vi "Real Time Display.vi"() -> ()   [LabVIEW 2015]
uses:
  Type/_Run Mode.ctl
  Type/_Data Operation.ctl
  Type/_RT Command.ctl
  Configuration/_Global Configuration.vi
  <vilib>/Utility/config.llb/Read Key (String).vi
  <vilib>/Utility/config.llb/Read Key (Double).vi
  <vilib>/Utility/config.llb/Read Key (I32).vi
  <vilib>/Utility/NIReport.llb/Append Image to Report (path wrap).vi
  <vilib>/Utility/NIReport.llb/NI_report.lvclass
  <vilib>/Utility/config.llb/NI_LVConfig.lvlib
panel:
  out "error out 2":errorcluster
  out "error out":errorcluster
  in  "Comments":string
  out "Close":bool
  out "Q2DC POL":bool
  out "Q1DC POL":bool
  out "Date":string
  out "MCA":bool
  out "Run Mode":T1
  out "Q2 Resolution":i32[](listbox) caption="Q2 +ve High Res"
  out "Q1 Resolution":i32[](listbox) caption="Q1 +ve High Res"
  out "Q2 Calibration":i32[](listbox)
  out "Q1 Calibration":i32[](listbox)
  out "Scan #":i32=1
  out "Peak List":i32[](listbox)
  out "Lens Values":i32[](listbox)
  out "TIC":cluster{"TIC X":dbl[], "TIC Y":dbl[]}[](graph)
  out "Run Time":i32=1 caption="Run Time (ms)"
  in  "Expt#":i32=1 caption="Experiment #"
  out "Init":bool
  out "A 6":bool
  out "A 5":bool
  out "A 4":bool
  out "A 3":bool
  out "A 2":bool
  out "A 1":bool
  out "MR 5":cluster{dbl[], dbl[]}(graph)
  out "MR 4":cluster{dbl[], dbl[]}(graph)
  out "MR 2":cluster{dbl[], dbl[]}(graph)
  out "MR 1":cluster{dbl[], dbl[]}(graph)
  out "MR 6":cluster{dbl[], dbl[]}(graph)
  out "MR 3":cluster{dbl[], dbl[]}(graph)
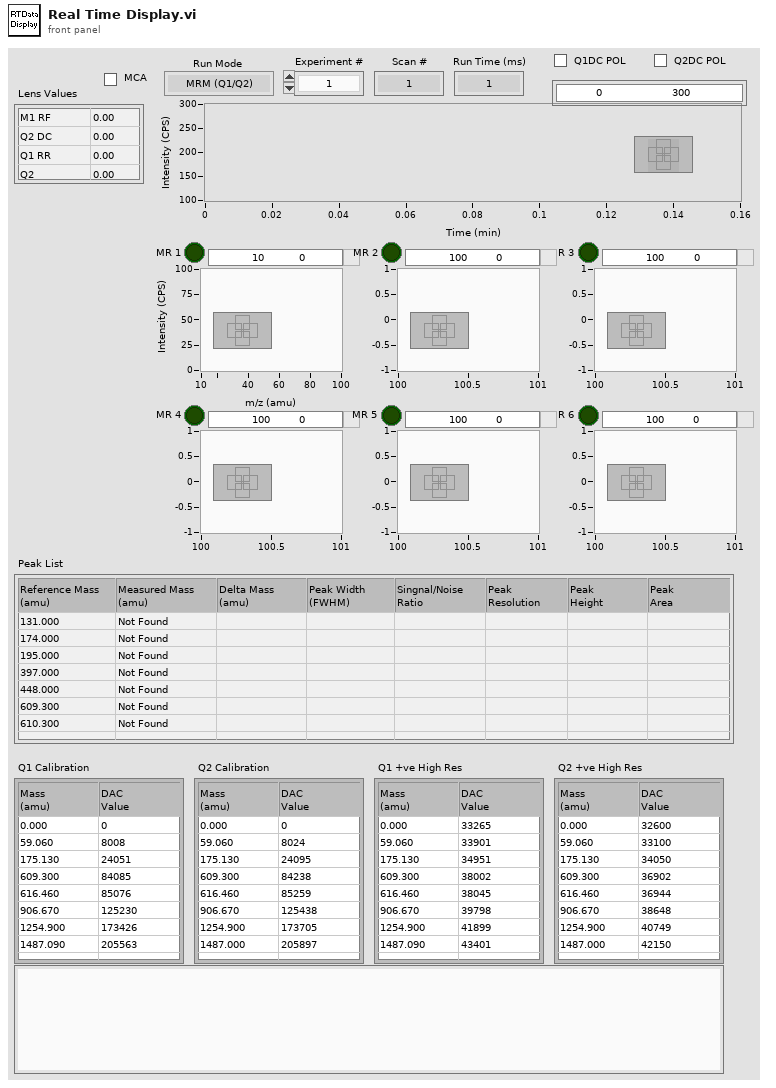
[diagram p1: front panel]
types:
  T1 = typedef "_Run Mode.ctl" = enum16{"MRM (Q1/Q2)", "Q1 Scan", "Q1 SRM", "Q2 Scan", "Q2 SRM", "Product Scan", "Precursor Scan", "Neutral Loss", "Neutral Gain"}
  T2 = cluster{"TIC":refnum<vi>, "MR 1":refnum<vi>, "MR 2":refnum<vi>, "MR 3":refnum<vi>, "MR 4":refnum<vi>, "MR 5":refnum<vi>, "MR 6":refnum<vi>, "A 1":refnum<vi>, "A 2":refnum<vi>, "A 3":refnum<vi>, "A 4":refnum<vi>, "A 5":refnum<vi>, "A 6":refnum<vi>, "Lens Values":refnum<vi>, "Q1 Calibration":refnum<vi>, "Q2 Calibration":refnum<vi>, "Q1 Resolution":refnum<vi>, "Q2 Resolution":refnum<vi>, "Peak List":refnum<vi>, "Comments":refnum<vi>}
  T3 = cluster{"RefMass":dbl[], "LensList":i32[], "SearchWin":dbl, "MinH":dbl, "MinW":i32, "RunTime":i32}
  T4 = enum16{"Standard Report", "HTML", "Word", "Excel"}
  T5 = typedef "_Data Operation.ctl" = enum8{"Initialize", "Get Data", "Set Data", "Close"}
  T6 = typedef "_RT Command.ctl" = enum16{"xml Start Run", "xml Start Actual Run", "xml Stop Run", "xml Runtime Update", "xml Get Status", "xml Get Table", "xml Set Table", "xml Get Configuration", "xml System Status", "xml Set LC Input Logic", "xml Get Data", "xml Get Info", "Start", "StartActualRun", "Stop", "Runtime Update", "Get Data", "Get Info", "Get Status", "Get Param", "Get Config", "Get Table", "Read ADC", "Set Oscillator", "Update Config", "Update Table", "Set All Pol", "Set Pol and DC", "Set Max Mass", "Toggle RP", "Toggle EL", "Set PIC", "Initialize Turbo", "Send Turbo Comm", "Close Turbo", "P1", "P2", "P3", "Send Serial", "Set LC Out", "Get LC In", "Read VAC", "Test Table", "Toggle Power", "Get Startup", "Set Startup", "Get ADC Table", "Set ADC Table", "Get Brief Status", "Get Detail Status", "Auxiliary Update", "Set CC Logics", "Set CC Input Logics", "Ignore Error", "invalid"}
  T7 = typedef "NI_LVConfig.lvlib/Config Data RefNum.ctl" = refnum<k1>
  T8 = typedef "_Current Data.ctl" = cluster{"Scan#":i32, "Run Time (mS)":i32, "TIC X":dbl[], "TIC Y":dbl[][], "MassRange":cluster{"X Title":string, "X":dbl[], "Y":i32[]}[], "Fixed Mass (amu)":dbl, "Method":T9}
  T9 = typedef "_XML Expt.ctl" = cluster{"StartT(mS)":i32, "#Cycles":i32, "PauseT(uS)":i32, "ScanType":i32, "Polarity":u8, "FixedMass":dbl, "DelayT(mS)":i32, "Active Ch":T10[], "Mass Range":T11[]}
  T10 = typedef "_XML Lens.ctl" = cluster{"Value":dbl, "ChID":u8}
  T11 = typedef "_Mass Range Property.ctl" = cluster{"Start":dbl, "Stop":dbl, "Step Size":dbl, "Steps":i32, "Dwell":dbl, "Parameters":T12[], "Res":T13}
  T12 = typedef "_Mass Range Parameters.ctl" = cluster{"Name":string, "Ch#":u8, "StartV":dbl, "StopV":dbl, "StepV":dbl, "Index":u8}
  T13 = typedef "_RT Res Type.ctl" = u16
  T14 = typedef "_Peak Property.ctl" = cluster{"Centroid":dbl, "Height":dbl, "FWHM":dbl, "Resolution":dbl, "Area":dbl, "StoN":dbl, "ApexX":dbl, "Baseline":dbl, "LEdgeX":dbl, "LEdgeY":dbl, "REdgeX":dbl, "REdgeY":dbl, "LEdgeFWHM":dbl, "REdgeFWHM":dbl}
  T15 = typedef "imagedata.ctl" = cluster{"image type":i32, "image depth":i32, "image":u8[], "mask":u8[], "colors":u32[], "Rectangle":cluster{"left":i16, "top":i16, "right":i16, "bottom":i16}}
  T16 = typedef "LVRangeTypeDef.ctl" = cluster{"Minimum":dbl, "Maximum":dbl, "Increment":dbl, "Minor Increment":dbl, "Start":dbl}
  T17 = typedef "LVPointDoubleTypeDef.ctl" = cluster{"Cursor X":dbl, "Cursor Y":dbl}
  T18 = cluster{"YScale.NameLbl.Text":string, "XScale.NameLbl.Text":string, "XScale.Range":T16, "YScale.Range":T16, "Label.Text":string, "Cursor.Cursor Position":T17, "Plot.Bar Plot Style":u8}
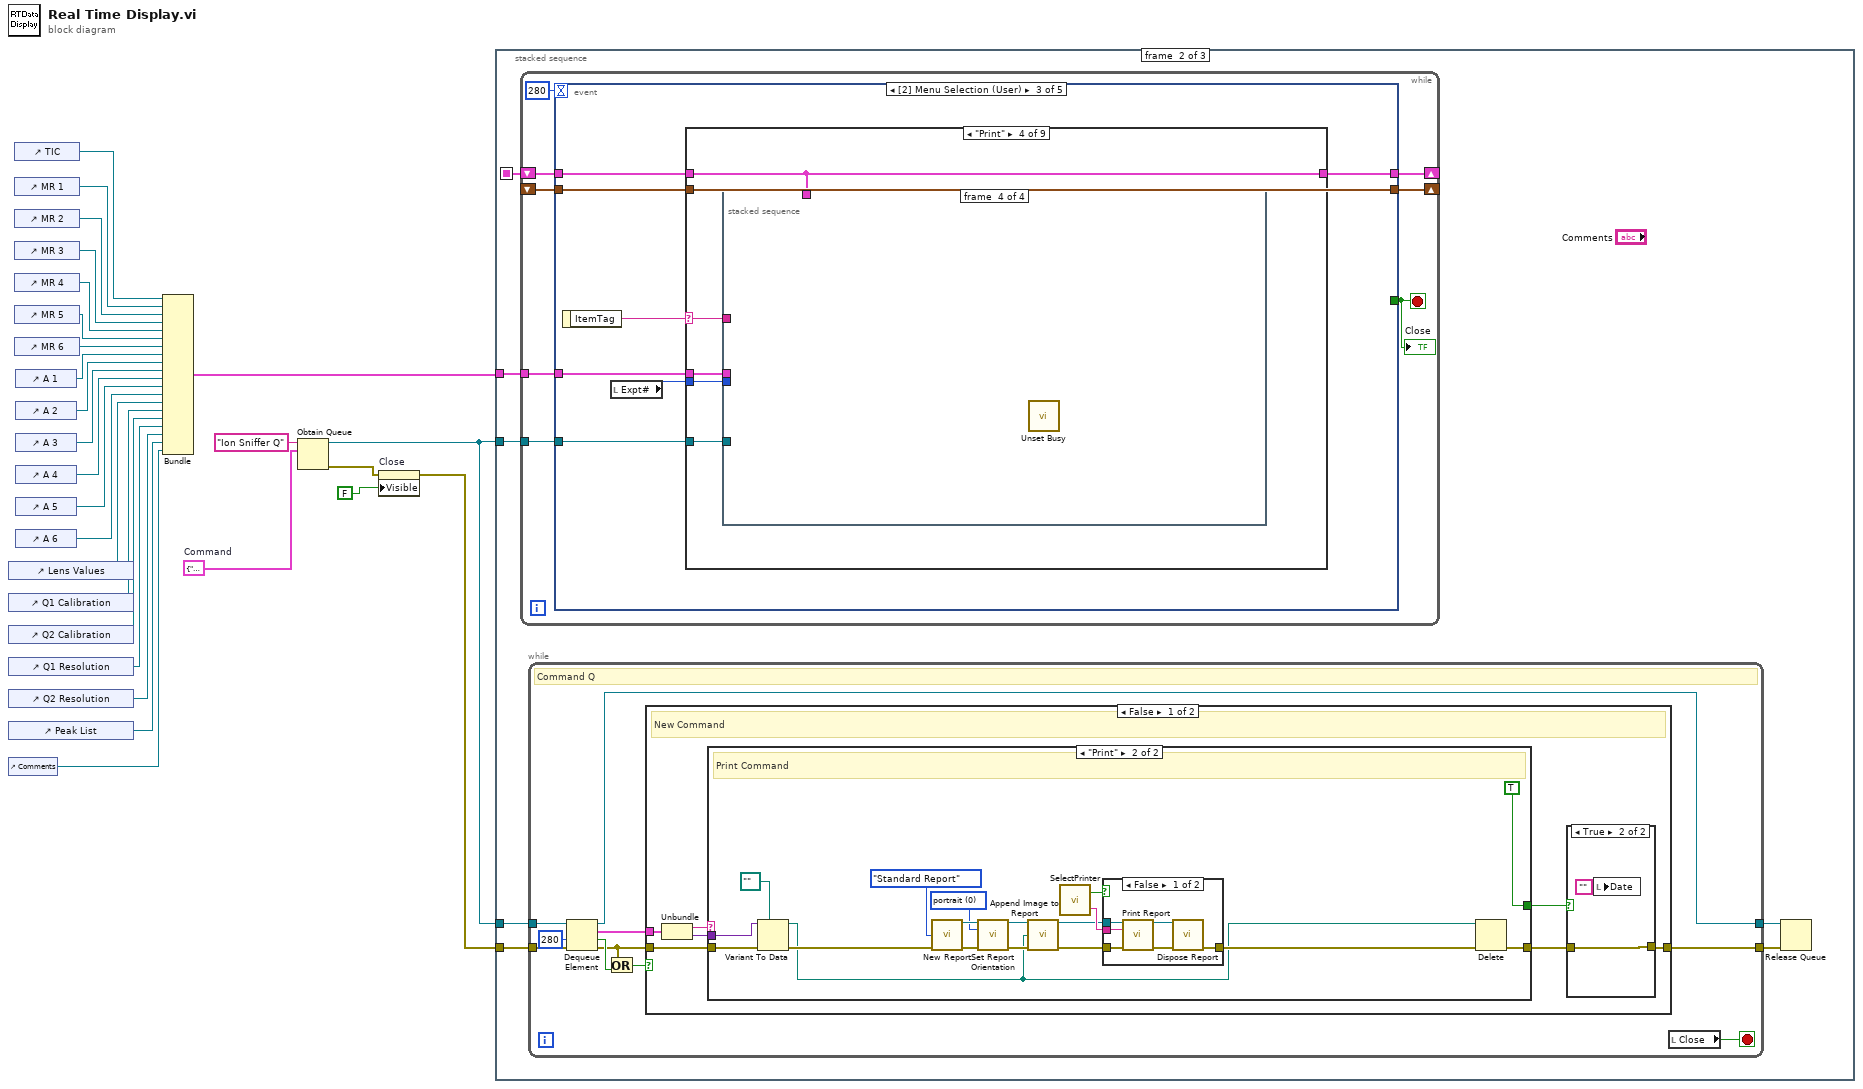
[diagram p0: block diagram]
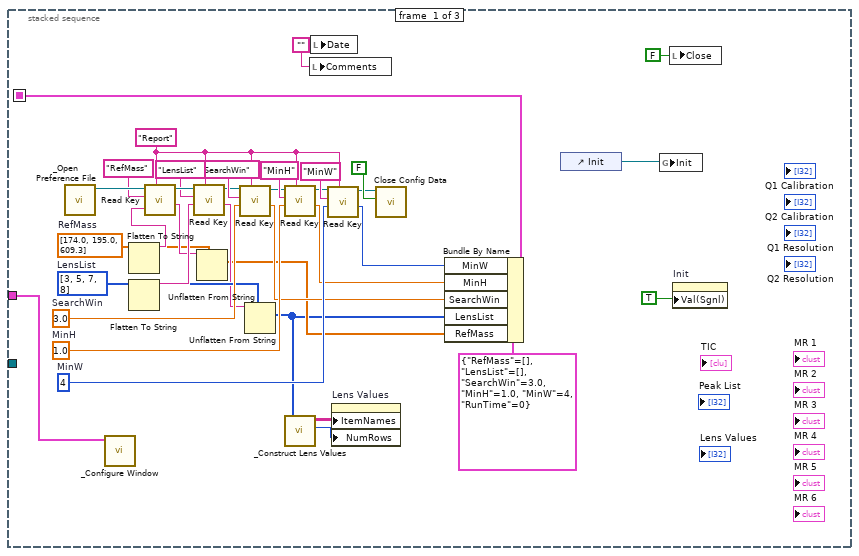
[diagram p2: hidden frame]
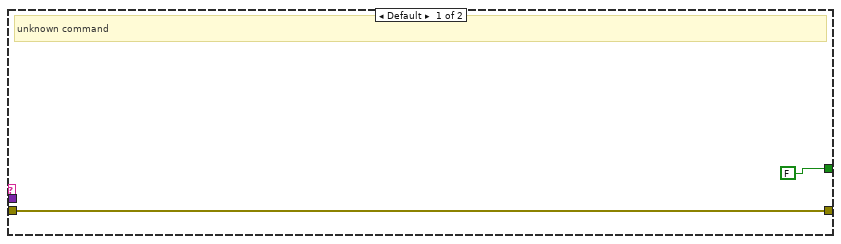
[diagram p4: hidden frame]
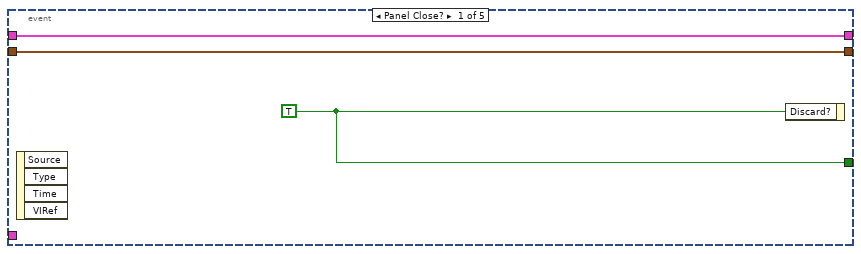
[diagram p7: hidden frame]
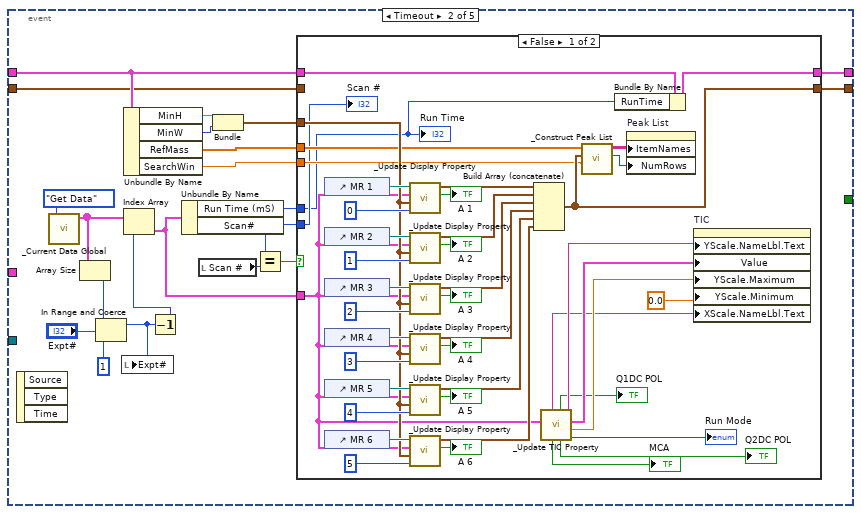
[diagram p8: hidden frame]
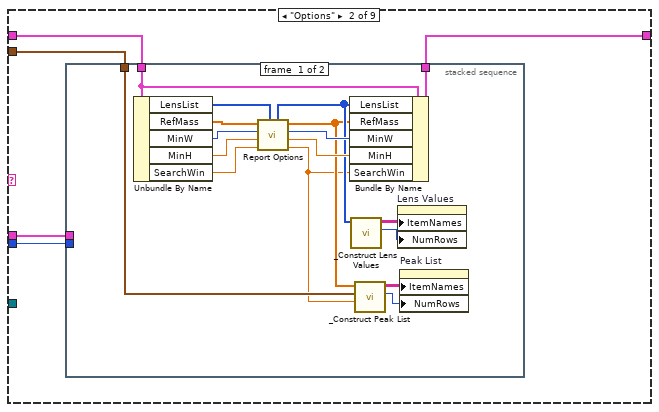
[diagram p11: hidden frame]
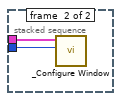
[diagram p12: hidden frame]
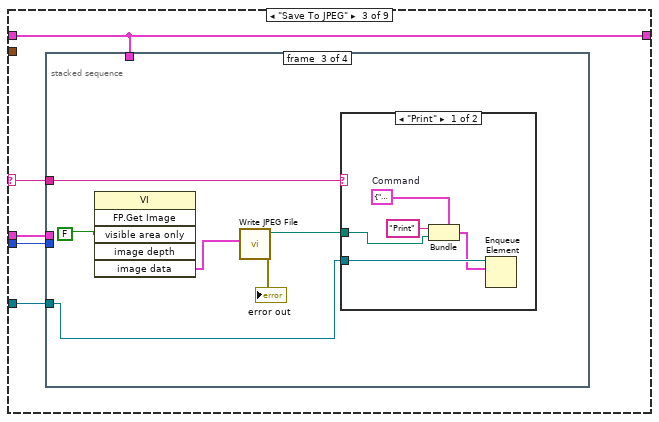
[diagram p13: hidden frame]
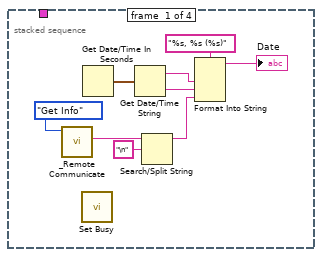
[diagram p14: hidden frame]
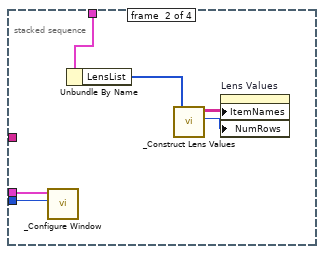
[diagram p15: hidden frame]
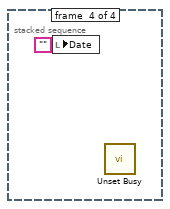
[diagram p17: hidden frame]
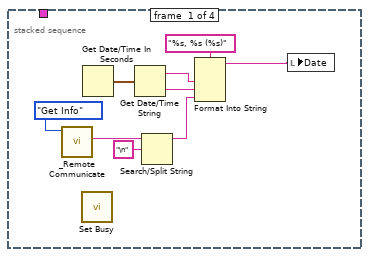
[diagram p18: hidden frame]
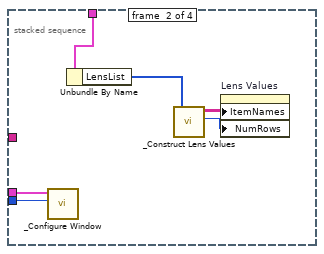
[diagram p19: hidden frame]
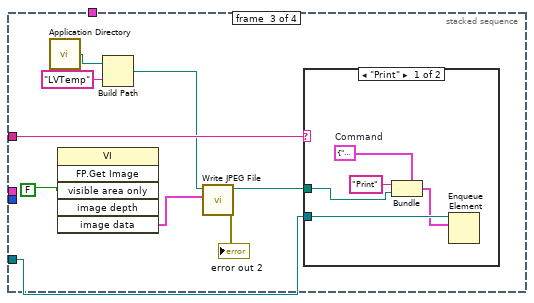
[diagram p20: hidden frame]
diagram:
  w1 = cluster{"Command":string, "Data":variant} {"Command"="", "Data"=variant}  # Command
  n1 = control-ref of="Lens Values"() -> (w27:refnum<vi>)
  n2 = control-ref of="Q1 Calibration"() -> (w13:refnum<vi>)
  n3 = control-ref of="Q2 Calibration"() -> (w12:refnum<vi>)
  n4 = control-ref of="Q1 Resolution"() -> (w11:refnum<vi>)
  n5 = control-ref of="Q2 Resolution"() -> (w10:refnum<vi>)
  n6 = control-ref of="Peak List"() -> (w9:refnum<vi>)
  n7 = control-ref of="Comments"() -> (w2:refnum<vi>)
  n8 = control-ref of="TIC"() -> (w8:refnum<vi>)
  n9 = control-ref of="MR 1"() -> (w15:refnum<vi>)
  n10 = control-ref of="MR 2"() -> (w16:refnum<vi>)
  n11 = control-ref of="MR 3"() -> (w17:refnum<vi>)
  n12 = control-ref of="MR 4"() -> (w18:refnum<vi>)
  n13 = control-ref of="MR 5"() -> (w19:refnum<vi>)
  n14 = control-ref of="MR 6"() -> (w20:refnum<vi>)
  n15 = control-ref of="A 1"() -> (w21:refnum<vi>)
  n16 = control-ref of="A 2"() -> (w22:refnum<vi>)
  n17 = control-ref of="A 3"() -> (w23:refnum<vi>)
  n18 = control-ref of="A 4"() -> (w24:refnum<vi>)
  n19 = control-ref of="A 5"() -> (w25:refnum<vi>)
  n20 = control-ref of="A 6"() -> (w26:refnum<vi>)
  n21 = Bundle("TIC"=w8, "MR 1"=w15, "MR 2"=w16, "MR 3"=w17, "MR 4"=w18, "MR 5"=w19, "MR 6"=w20, "A 1"=w21, "A 2"=w22, "A 3"=w23, "A 4"=w24, "A 5"=w25, "A 6"=w26, "Lens Values"=w27, "Q1 Calibration"=w13, "Q2 Calibration"=w12, "Q1 Resolution"=w11, "Q2 Resolution"=w10, "Peak List"=w9, "Comments"=w2) -> (w14:T2)  [unwired: 1 out]
  n22 = Obtain Queue(name (unnamed)="Ion Sniffer Q", element data type=w1) -> (queue out=w6:refnum<queue>, error out=w4:errorcluster)  [unwired: 3 in, 1 out]
  n23 = property on="Close" class="Bool (strict)"(error in=w4, "Visible"=FALSE) -> (error out=w5:errorcluster)  [unwired: 1 in, 1 out]
  n24 = stacked-sequence {
    seq-local: [w34 _ _] -> [_ w70 _]
    tunnel: w14 -> [w30 w69 _]
    tunnel: w6 -> [_ w68 _]
    tunnel: w6 -> [_ w67 _]
    tunnel: w5 -> [_ w66 _]
    frame #0 {
      w28 = ""
      w50 = "Report" ("section")
      w41 = i32[] [3, 5, 7, 8]  # LensList
      w46 = 4  # MinW
      w47 = 1.0  # MinH
      w48 = 3.0  # SearchWin
      w42 = dbl[] [174.0, 195.0, 609.3]  # RefMass
      n25 = call "_Open Preference File.vi"() -> ("refnum"=w59:T7)  [unwired: 3 in, 4 out]
      n26 = call "_Configure Window.vi"("ControlRef"=w30) -> ()  [unwired: 2 in, 5 out]
      n27 = Flatten To String(anything=w42) -> (data string=w45:string)  [unwired: 1 in, 4 out]
      n28 = Flatten To String(anything=w41) -> (data string=w44:string)  [unwired: 1 in, 4 out]
      n29 = call-poly <vilib>:"Read Key.vi"("section"=w50, "default value"=w45, "key"="RefMass", "refnum"=w59) -> ("value"=w43:string, "refnum out"=w61:T7)  [unwired: 2 in, 4 out]
      n30 = call-poly <vilib>:"Read Key.vi"("section"=w50, "default value"=w44, "key"="LensList" ("section"), "refnum"=w61) -> ("value"=w40:string, "refnum out"=w53:T7)  [unwired: 2 in, 4 out]
      n31 = Unflatten From String(type=w42, binary string=w43) -> (value=w35:dbl[])  [unwired: 1 in, 4 out]
      n32 = call-poly <vilib>:"Read Key.vi"("section"=w50, "default value"=w48, "key"="SearchWin", "refnum"=w53) -> ("value"=w36:dbl, "refnum out"=w54:T7)  [unwired: 1 in, 5 out]
      n33 = Unflatten From String(type=w41, binary string=w40) -> (value=w33:i32[])  [unwired: 1 in, 4 out]
      n34 = call-poly <vilib>:"Read Key.vi"("section"=w50, "default value"=w47, "key"="MinH" ("section"), "refnum"=w54) -> ("value"=w37:dbl, "refnum out"=w51:T7)  [unwired: 1 in, 5 out]
      n35 = call "_Construct Lens Values.vi"("Lens List"=w33) -> ("# of Lens"=w31:i32, "Table"=w32:string[][])  [unwired: 5 out]
      n36 = local write "Comments"(w28) -> ()
      n37 = local write "Date"(w28) -> ()
      n38 = call-poly <vilib>:"Read Key.vi"("section"=w50, "default value"=w46, "key"="MinW" ("section"), "refnum"=w51) -> ("value"=w38:i32, "refnum out"=w49:T7)  [unwired: 1 in, 5 out]
      n39 = property on="Lens Values" class="MCListbox (strict)"("ItemNames"=w32, "NumRows"=w31) -> ()  [unwired: 2 in, 2 out]
      n40 = call <vilib>:"Close Config Data.vi"("write file if changed (T)"=FALSE ("write configuration file? (F)"), "refnum"=w49) -> ()  [unwired: 1 in, 9 out]
      n41 = Bundle By Name(cluster=T3 {"RefMass"=[], "LensList"=[], "SearchWin"=3.0, "MinH"=1.0, "MinW"=4, "RunTime"=0}, "MinW"=w38, "MinH"=w37, "SearchWin"=w36, "LensList"=w33, "RefMass"=w35) -> (w34:T3)
      n42 = control-ref of="Init"() -> (w63:refnum<vi>)
      n43 = global write "_Global Configuration.vi" "Init"(w63) -> ()
      n44 = local write "Close"(FALSE ("Close")) -> ()
      n45 = property on="Init" class="Bool (strict)"("Val(Sgnl)"=TRUE ("Value (Signaling)")) -> ()  [unwired: 2 in, 2 out]
    }
    frame #1 {
      n46 = while {
        shift-right: [w125] -> _
        shift-left: w70 -> [w126]
        shift-right: [w124] -> _
        shift-left: _ -> [w123]
        tunnel: w69 -> [w122]
        tunnel: w68 -> [w120]
        stop <- w119 stop-if-true
        n47 = event shown="[2] Menu Selection (User)" {
          selector: _ -> [_ _ _ _ _]
          dyn-events: _ -> [_ _ _ _ _]
          timeout: 280 -> [_ _ _ _ _]
          tunnel: [w129 _ _ _ _] -> w119
          tunnel: w126 -> [w128 w150 w202 w322 w328]
          tunnel: [w128 w149 w201 w323 w328] -> w125
          tunnel: [w127 w147 w200 w318 w327] -> w124
          tunnel: w123 -> [w127 w148 w200 w318 w327]
          tunnel: w122 -> [_ _ w199 w316 _]
          tunnel: w120 -> [_ _ w197 _ _]
          event Panel Close? {
            w129 = TRUE ("Discard?")
            n48 = event-data() -> ()  [unwired: 5 out]
            n49 = event-data("Discard?"=w129) -> ()  [unwired: 1 in, 1 out]
          }
          event Timeout {
            n50 = event-data() -> ()  [unwired: 4 out]
            n51 = call "_Current Data Global.vi"("Operation"=_Data_Operation."Get Data") -> ("CurrentData"=w139:T8[])  [unwired: 3 in, 3 out]
            n52 = Array Size(array=w139) -> (size(s)=w136:i32)
            n53 = In Range and Coerce(upper limit=w136, x="Expt#", lower limit=1) -> (coerced(x)=w135:i32)  [unwired: 1 out]
            n54 = local write "Expt#"(w135) -> ()
            n55 = Unbundle By Name(w150) -> ("MinH"=w145:dbl, "MinW"=w144:i32, "RefMass"=w142:dbl[], "SearchWin"=w141:dbl)
            n56 = Decrement(x=w135) -> (x-1=w134:i32)
            n57 = Index Array(array=w139, index=w134) -> (element=w140:T8)
            n58 = Unbundle By Name(w140) -> ("Run Time (mS)"=w130:i32, "Scan#"=w132:i32)
            n59 = local read "Scan #"() -> (w133:i32)
            n60 = Bundle("MinH"=w145, "MinW"=w144) -> (w143:cluster{"MinH":dbl, "MinW":i32})  [unwired: 1 out]
            n61 = Equal?(x=w132, y=w133) -> (x = y?=w131:bool)
            n62 = case shown="False" w131 {
              tunnel: w150 -> [w194 w196]
              tunnel: [w193 w196] -> w149
              tunnel: [w165 w195] -> w147
              tunnel: w148 -> [_ w195]
              tunnel: w143 -> [w179 _]
              tunnel: w140 -> [w161 _]
              tunnel: w142 -> [w164 _]
              tunnel: w141 -> [w163 _]
              tunnel: w132 -> [w162 _]
              tunnel: w130 -> [w154 _]
              frame False {
                n63 = control-ref of="MR 1"() -> (w192:refnum<vi>)
                n64 = control-ref of="MR 2"() -> (w191:refnum<vi>)
                n65 = control-ref of="MR 3"() -> (w189:refnum<vi>)
                n66 = control-ref of="MR 4"() -> (w187:refnum<vi>)
                n67 = control-ref of="MR 5"() -> (w185:refnum<vi>)
                n68 = control-ref of="MR 6"() -> (w183:refnum<vi>)
                n69 = call "_Update Display Property.vi"("MassRange# (0)"=0, "PeakParam"=w179, "Current Data"=w161, "Display Refnum"=w192) -> ("Active"=→"A 1":bool, "Peak List"=w173:T14[])  [unwired: 3 out]
                n70 = call "_Update Display Property.vi"("MassRange# (0)"=1, "PeakParam"=w179, "Current Data"=w161, "Display Refnum"=w191) -> ("Active"=→"A 2":bool, "Peak List"=w172:T14[])  [unwired: 3 out]
                n71 = call "_Update Display Property.vi"("MassRange# (0)"=2, "PeakParam"=w179, "Current Data"=w161, "Display Refnum"=w189) -> ("Active"=→"A 3":bool, "Peak List"=w171:T14[])  [unwired: 3 out]
                n72 = call "_Update Display Property.vi"("MassRange# (0)"=3, "PeakParam"=w179, "Current Data"=w161, "Display Refnum"=w187) -> ("Active"=→"A 4":bool, "Peak List"=w170:T14[])  [unwired: 3 out]
                n73 = call "_Update Display Property.vi"("MassRange# (0)"=4, "PeakParam"=w179, "Current Data"=w161, "Display Refnum"=w185) -> ("Active"=→"A 5":bool, "Peak List"=w169:T14[])  [unwired: 3 out]
                n74 = call "_Update Display Property.vi"("MassRange# (0)"=5, "PeakParam"=w179, "Current Data"=w161, "Display Refnum"=w183) -> ("Active"=→"A 6":bool, "Peak List"=w168:T14[])  [unwired: 3 out]
                n75 = Build Array (concatenate)(w173, w172, w171, w170, w169, w168) -> (w165:T14[])
                n76 = call "_Update TIC Property.vi"("Current Data"=w161) -> ("Run Mode"=→"Run Mode":T1, "YMax"=w158:dbl, "TIC Data"=w159:cluster{"TIC X":dbl[], "Data in cps":dbl[]}[], "YTitle"=w160:string, "Q2DC Pol"=→"Q2DC POL":bool, "Q1DC Pol"=→"Q1DC POL":bool, "MCA"=→"MCA":bool, "XTitle"=w153:string)  [unwired: 3 out]
                n77 = call "_Construct Peak List.vi"("Search Window"=w163, "Peak List"=w165, "RefMass"=w164) -> ("# of Peaks"=w166:i32, "Table"=w167:string[][])  [unwired: 3 out]
                n78 = Bundle By Name(cluster=w194, "RunTime"=w154) -> (w193:T3)
                n79 = property on="Peak List" class="MCListbox (strict)"("ItemNames"=w167, "NumRows"=w166) -> ()  [unwired: 2 in, 2 out]
                n80 = property on="TIC" class="XYGraph (strict)"("YScale.NameLbl.Text"=w160, "Value"=w159, "YScale.Maximum"=w158, "YScale.Minimum"=0.0 ("Y Scale.Range:Minimum"), "XScale.NameLbl.Text"=w153) -> ()  [unwired: 2 in, 2 out]
                "Run Time" <- w154
                "Scan #" <- w162
              }
              frame True {
              }
            }
          }
          event Menu Selection (User) {
            n81 = event-data() -> ("ItemTag"=w203:string)  [unwired: 1 out]
            n82 = local read "Expt#"() -> (w198:i32)
            n83 = case shown="\"Print\"" w203 {
              selector: w203 -> [_ _ w230 w262 _ _ _ _ _]
              tunnel: w202 -> [w204 w209 w233 w265 w297 w298 w301 w303 w315]
              tunnel: [w204 w208 w233 w265 w297 w298 w301 w303 w315] -> w201
              tunnel: w200 -> [_ w207 _ _ w296 _ _ _ _]
              tunnel: w199 -> [_ w206 w232 w264 _ _ _ w304 w314]
              tunnel: w198 -> [_ w205 w231 w263 _ _ _ w302 w313]
              tunnel: w197 -> [_ _ w229 w261 _ _ _ _ _]
              frame Default {
              }
              frame "Options" {
                n84 = stacked-sequence {
                  tunnel: w209 -> [w210 _]
                  tunnel: [w221 _] -> w208
                  tunnel: w207 -> [w218 _]
                  tunnel: w206 -> [_ w228]
                  tunnel: w205 -> [_ w227]
                  frame #0 {
                    n85 = Unbundle By Name(w210) -> ("LensList"=w226:i32[], "RefMass"=w217:dbl[], "MinW"=w225:i32, "MinH"=w224:dbl, "SearchWin"=w216:dbl)
                    n86 = call "Report Options.vi"("LensList"=w226, "Search Window"=w216, "Min. Height"=w224, "Min. Width"=w225, "RefMass"=w217) -> ("Search Window 2"=w211:dbl, "Min. Height 2"=w222:dbl, "Min. Width 2"=w223:i32, "RefMass 2"=w212:dbl[], "LensList 2"=w213:i32[])
                    n87 = Bundle By Name(cluster=w210, "LensList"=w213, "RefMass"=w212, "MinW"=w223, "MinH"=w222, "SearchWin"=w211) -> (w221:T3)
                    n88 = call "_Construct Lens Values.vi"("Lens List"=w213) -> ("# of Lens"=w214:i32, "Table"=w215:string[][])  [unwired: 5 out]
                    n89 = call "_Construct Peak List.vi"("Search Window"=w211, "Peak List"=w218, "RefMass"=w212) -> ("# of Peaks"=w219:i32, "Table"=w220:string[][])  [unwired: 3 out]
                    n90 = property on="Lens Values" class="MCListbox (strict)"("ItemNames"=w215, "NumRows"=w214) -> ()  [unwired: 2 in, 2 out]
                    n91 = property on="Peak List" class="MCListbox (strict)"("ItemNames"=w220, "NumRows"=w219) -> ()  [unwired: 2 in, 2 out]
                  }
                  frame #1 {
                    n92 = call "_Configure Window.vi"("Expt#"=w227, "ControlRef"=w228) -> ()  [unwired: 1 in, 5 out]
                  }
                }
              }
              frame "Save To JPEG" {
                n93 = stacked-sequence {
                  tunnel: w233 -> [_ w246 _ _]
                  tunnel: w232 -> [_ w244 _ _]
                  tunnel: w231 -> [_ w243 _ _]
                  tunnel: w230 -> [_ _ w252 _]
                  tunnel: w229 -> [_ _ w249 _]
                  frame #0 {
                    n94 = call "_Remote Communicate.vi"("Command"=_RT_Command."Get Info") -> ("Info"=w241:string)  [unwired: 5 in, 3 out]
                    n95 = call <vilib>:"Set Busy.vi"() -> ()  [unwired: 4 in, 8 out]
                    n96 = Get Date/Time In Seconds() -> (seconds since 1Jan1904=w239:timestamp)
                    n97 = Get Date/Time String(seconds (now)=w239) -> (date string=w237:string, time string=w236:string)  [unwired: 2 out]
                    n98 = Search/Split String(string=w241, search string/char (-)="\n") -> (substring before match=w235:string)  [unwired: 3 out]
                    n99 = Format Into String(format string="%s, %s (%s)", w237, w236, w235) -> (resulting string=→"Date":string)  [unwired: 2 in, 1 out]
                  }
                  frame #1 {
                    n100 = call "_Configure Window.vi"("Expt#"=w243, "ControlRef"=w244) -> ()  [unwired: 1 in, 5 out]
                    n101 = Unbundle By Name(w246) -> ("LensList"=w245:i32[])
                    n102 = call "_Construct Lens Values.vi"("Lens List"=w245) -> ("# of Lens"=w247:i32, "Table"=w248:string[][])  [unwired: 5 out]
                    n103 = property on="Lens Values" class="MCListbox (strict)"("ItemNames"=w248, "NumRows"=w247) -> ()  [unwired: 2 in, 2 out]
                  }
                  frame #2 {
                    n104 = invoke class="VI" method="FP.Get Image"("visible area only"=FALSE ("Visible Area Only")) -> ("image data"=w253:T15)  [unwired: 5 in, 5 out]
                    n105 = call <vilib>:"Write JPEG File.vi"("image data"=w253) -> ("error out"=→"error out":errorcluster, "path"=w251:path)  [unwired: 2 in, 7 out]
                    n106 = case shown="\"Print\"" w252 {
                      tunnel: w251 -> [w255 _]
                      tunnel: w249 -> [w259 _]
                      frame "Print" {
                        w258 = cluster{"Command":string, "Data":variant} {"Command"="", "Data"=variant}  # Command
                        n107 = Bundle(cluster=w258, "Command"="Print", "Data"=w255) -> (w256:cluster{"Command":string, "Data":variant})
                        n108 = Enqueue Element(queue=w259, element=w256) -> ()  [unwired: 2 in, 3 out]
                      }
                      frame Default {
                      }
                    }
                  }
                  frame #3 {
                    n109 = local write "Date"("") -> ()
                    n110 = call <vilib>:"Unset Busy.vi"() -> ()  [unwired: 2 in, 10 out]
                  }
                }
              }
              frame "Print" {
                n111 = stacked-sequence {
                  tunnel: w265 -> [_ w278 _ _]
                  tunnel: w264 -> [_ w276 _ _]
                  tunnel: w263 -> [_ w275 _ _]
                  tunnel: w262 -> [_ _ w287 _]
                  tunnel: w261 -> [_ _ w284 _]
                  frame #0 {
                    n112 = call "_Remote Communicate.vi"("Command"=_RT_Command."Get Info") -> ("Info"=w273:string)  [unwired: 5 in, 3 out]
                    n113 = call <vilib>:"Set Busy.vi"() -> ()  [unwired: 4 in, 8 out]
                    n114 = Get Date/Time In Seconds() -> (seconds since 1Jan1904=w271:timestamp)
                    n115 = Get Date/Time String(seconds (now)=w271) -> (date string=w269:string, time string=w268:string)  [unwired: 2 out]
                    n116 = Search/Split String(string=w273, search string/char (-)="\n") -> (substring before match=w267:string)  [unwired: 3 out]
                    n117 = Format Into String(format string="%s, %s (%s)", w269, w268, w267) -> (resulting string=w266:string)  [unwired: 2 in, 1 out]
                    n118 = local write "Date"(w266) -> ()
                  }
                  frame #1 {
                    n119 = call "_Configure Window.vi"("Expt#"=w275, "ControlRef"=w276) -> ()  [unwired: 1 in, 5 out]
                    n120 = Unbundle By Name(w278) -> ("LensList"=w277:i32[])
                    n121 = call "_Construct Lens Values.vi"("Lens List"=w277) -> ("# of Lens"=w279:i32, "Table"=w280:string[][])  [unwired: 5 out]
                    n122 = property on="Lens Values" class="MCListbox (strict)"("ItemNames"=w280, "NumRows"=w279) -> ()  [unwired: 2 in, 2 out]
                  }
                  frame #2 {
                    n123 = call <vilib>:"Application Directory.vi"() -> ("Application Directory"=w283:path)
                    n124 = invoke class="VI" method="FP.Get Image"("visible area only"=FALSE ("Visible Area Only")) -> ("image data"=w288:T15)  [unwired: 5 in, 5 out]
                    n125 = Build Path(base path=w283, name or relative path="LVTemp") -> (appended path=w281:path)
                    n126 = call <vilib>:"Write JPEG File.vi"("image data"=w288, "path to JPEG file"=w281) -> ("error out"=→"error out 2":errorcluster, "path"=w286:path)  [unwired: 1 in, 7 out]
                    n127 = case shown="\"Print\"" w287 {
                      tunnel: w286 -> [w290 _]
                      tunnel: w284 -> [w294 _]
                      frame "Print" {
                        w293 = cluster{"Command":string, "Data":variant} {"Command"="", "Data"=variant}  # Command
                        n128 = Bundle(cluster=w293, "Command"="Print", "Data"=w290) -> (w291:cluster{"Command":string, "Data":variant})
                        n129 = Enqueue Element(queue=w294, element=w291) -> ()  [unwired: 2 in, 3 out]
                      }
                      frame Default {
                      }
                    }
                  }
                  frame #3 {
                    n130 = call <vilib>:"Unset Busy.vi"() -> ()  [unwired: 2 in, 10 out]
                  }
                }
              }
              frame "List All Peaks" {
                n131 = call "Display Data List.vi"("Peak List"=w296, "Data Type"=enum16{"TIC", "Spectrum", "Peak"}."Peak") -> ()  [unwired: 8 out]
              }
              frame "List TIC Data" {
                n132 = call "Display Data List.vi"("Data Type"=enum16{"TIC", "Spectrum", "Peak"}."TIC") -> ()  [unwired: 3 in, 6 out]
              }
              frame "List Spectral Data" {
                n133 = call "Display Data List.vi"("Data Type"=enum16{"TIC", "Spectrum", "Peak"}."Spectrum") -> ()  [unwired: 1 in, 8 out]
              }
              frame "Show Lens Values" {
                n134 = flat-sequence {
                  tunnel: w304 -> [w306]
                  tunnel: w302 -> [w305]
                  tunnel: w303 -> [w308]
                  frame #0 {
                    n135 = call "_Configure Window.vi"("For Printing (T)"=TRUE ("For Printing (F)"), "Expt#"=w305, "ControlRef"=w306) -> ()  [unwired: 5 out]
                  }
                  frame #1 {
                    n136 = Unbundle By Name(w308) -> ("LensList"=w309:i32[])
                    n137 = call "_Construct Lens Values.vi"("Lens List"=w309) -> ("# of Lens"=w310:i32, "Table"=w311:string[][])  [unwired: 5 out]
                    n138 = property on="Lens Values" class="MCListbox (strict)"("ItemNames"=w311, "NumRows"=w310) -> ()  [unwired: 2 in, 2 out]
                  }
                }
              }
              frame "Hide Lens Values" {
                n139 = call "_Configure Window.vi"("For Printing (T)"=FALSE, "Expt#"=w313, "ControlRef"=w314) -> ()  [unwired: 5 out]
              }
            }
          }
          event "Init": Value Change {
            w317 = 0 ("RunTime")
            # "This event must be sent at the start of each run"
            n140 = event-data() -> ()  [unwired: 7 out]
            n141 = Unbundle By Name(w322) -> ("LensList"=w319:i32[])
            n142 = call "_Configure Window.vi"("ControlRef"=w316) -> ()  [unwired: 2 in, 5 out]
            n143 = call "_Construct Lens Values.vi"("Lens List"=w319) -> ("# of Lens"=w320:i32, "Table"=w321:string[][])  [unwired: 5 out]
            n144 = property on="Lens Values" class="MCListbox (strict)"("ItemNames"=w321, "NumRows"=w320) -> ()  [unwired: 2 in, 2 out]
            n145 = Bundle By Name(cluster=w322, "RunTime"=w317) -> (w323:T3)
            n146 = local write "Scan #"(w317) -> ()
            n147 = local write "Run Time"(w317) -> ()
            "Init" <- FALSE ("Init")
          }
          event "MR 1", "MR 2", "MR 3", "MR 4", "MR 5", "MR 6", "TIC": Mouse Down? {
            n148 = event-data() -> ("CtlRef"=w325:refnum<vi>, "Mods.Double Click"=w326:bool)  [unwired: 4 out]
            n149 = case shown="True" w326 {
              tunnel: w325 -> [_ w343]
              frame False {
              }
              frame True {
                n150 = call "_Launch Dynamic VI.vi"("VI Name"=path "Show One Plot.vi" ("name or relative path")) -> ("VI Refnum"=w345:refnum<vi>)  [unwired: 3 out]
                n151 = property class="XYGraph"(reference=w343) -> ("YScale.NameLbl.Text"=w341:string, "XScale.NameLbl.Text"=w340:string, "XScale.Range"=w339:T16, "YScale.Range"=w338:T16, "Label.Text"=w337:string, "Cursor.Cursor Position"=w336:T17, "Plot.Bar Plot Style"=w329:u8)  [unwired: 1 in, 2 out]
                n152 = property class="VI"(reference=w345) -> (reference out=w348:refnum<vi>, error out=w347:errorcluster, "Front Panel"=w346:refnum<vi>)  [unwired: 1 in]
                n153 = property class="Pnl"(reference=w346, error in=w347) -> (error out=w334:errorcluster, "Controls[]"=w335:refnum<vi>[])  [unwired: 1 out]
                n154 = Bundle("YScale.NameLbl.Text"=w341, "XScale.NameLbl.Text"=w340, "XScale.Range"=w339, "YScale.Range"=w338, "Label.Text"=w337, "Cursor.Cursor Position"=w336, "Plot.Bar Plot Style"=w329) -> (w331:T18)  [unwired: 1 out]
                n155 = To Variant(anything=w331) -> (Variant=w330:variant)
                n156 = call "_Get Server Control.vi"("error in (no error)"=w334, "Control Name"="Data", "All Controls[]"=w335) -> ("error out"=w342:errorcluster, "Ctl Refnum"=w332:refnum<vi>)  [unwired: 3 out]
                n157 = property class="Ctl"(reference=w332, "Val(Sgnl)"=w330) -> ()  [unwired: 1 in, 2 out]
                n158 = Close Reference(reference=w348, error in (no error)=w342) -> ()  [unwired: 1 out]
              }
            }
            n159 = event-data() -> ()  [unwired: 1 in, 5 out]
          }
        }
        "Close" <- w119
      }
      n160 = while {
        tunnel: w67 -> [w79]
        tunnel: w66 -> [w80]
        tunnel: [w76] -> w64
        tunnel: [w75] -> w65
        stop <- w71 stop-if-true
        # "Command Q"
        n161 = Dequeue Element(queue=w79, timeout in ms (-1)=280, error in (no error)=w80) -> (queue out=w75:refnum<queue>, element=w78:cluster{"Command":string, "Data":variant}, timed out?=w74:bool, error out=w73:errorcluster)
        n162 = Or(x=w73, y=w74) -> (x .or. y?=w72:bool)
        n163 = case shown="False" w72 {
          tunnel: w73 -> [w84 w118]
          tunnel: w78 -> [w87 _]
          tunnel: [w82 w118] -> w76
          frame False {
            # "New Command"
            n164 = Unbundle(w87) -> ("Command"=w85:string, "Data"=w86:variant)
            n165 = case shown="\"Print\"" w85 {
              tunnel: w86 -> [_ w108]
              tunnel: w84 -> [w92 w110]
              tunnel: [w92 w109] -> w83
              tunnel: [FALSE TRUE] -> w81
              frame Default {
                # "unknown command"
              }
              frame "Print" {
                w102 = 0 items=["portrait", "landscape"] ("orientation (portrait)")
                # "Print Command"
                n166 = Variant To Data(error in=w110, type=path "", Variant=w108) -> (data=w93:path, error out=w98:errorcluster)
                n167 = call <vilib>:"New Report.vi"("report type"=T4."Standard Report", "error in (no error)"=w98) -> ("report out"=w103:refnum<class "NI_report.lvclass">, "error out"=w97:errorcluster)  [unwired: 12 in]
                n168 = call-dynamic "Set Report Orientation.vi"("report in"=w103, "orientation (portrait)"=w102, "error in (no error)"=w97) -> ("report out"=w105:refnum<class "NI_report.lvclass">, "error out"=w96:errorcluster)  [unwired: 11 in]
                n169 = call-poly <vilib>:"Append Image to Report.vi"("report in"=w105, "path or URL of image"=w93, "error in (no error)"=w96) -> ("report out"=w99:refnum<class "NI_report.lvclass">, "error out"=w95:errorcluster)  [unwired: 9 in, 2 out]
                n170 = call "SelectPrinter.vi"() -> ("ChosenPrinter"=w100:string, "Closed?"=w101:bool)  [unwired: 2 in]
                n171 = case shown="False" w101 {
                  tunnel: w100 -> [w115 _]
                  tunnel: w95 -> [w114 w117]
                  tunnel: [w112 w117] -> w94
                  tunnel: w99 -> [w111 _]
                  frame False {
                    n172 = call-dynamic "Print Report.vi"("report in"=w111, "printer name (default)"=w115, "error in (no error)"=w114) -> ("report out"=w116:refnum<class "NI_report.lvclass">, "error out"=w113:errorcluster)  [unwired: 11 in]
                    n173 = call-dynamic "Dispose Report.vi"("report in"=w116, "error in (no error)"=w113) -> ("error out"=w112:errorcluster)  [unwired: 13 in]
                  }
                  frame True {
                  }
                }
                n174 = Delete(path (use dialog)=w93, error in=w94) -> (error out=w109:errorcluster)  [unwired: 3 in, 2 out]
              }
            }
            n175 = case shown="True" w81 {
              tunnel: [w88 w90] -> w82
              tunnel: w83 -> [w88 w90]
              frame False {
              }
              frame True {
                n176 = local write "Date"("") -> ()
              }
            }
          }
          frame True {
            # "Timeout/Error"
          }
        }
        n177 = local read "Close"() -> (w71:bool)
      }
      n178 = Release Queue(queue=w65, error in (no error)=w64) -> ()  [unwired: 1 in, 3 out]
    }
    frame #2 {
      n179 = property class="VI"("Front Panel.Open"=FALSE ("Front Panel Window:Open")) -> ()  [unwired: 2 in, 2 out]
    }
  }
